vi "PreferencesLoop.vi"   [LabVIEW 2013]
panel:
  # "Test Subsystem"
  # "Other Subsystem"
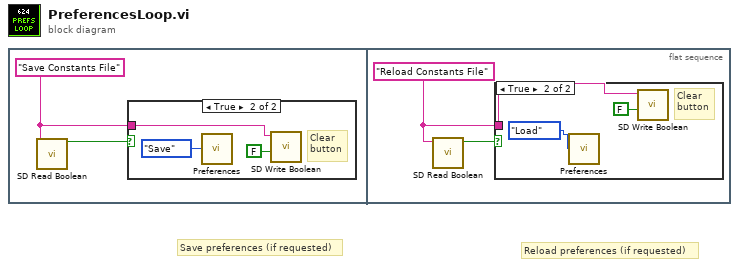
[diagram p0: block diagram]
diagram:
  # "Reload preferences (if requested)"
  # "Save preferences (if requested)"
  n1 = flat-sequence {
    frame #0 {
      w1 = "Save Constants File" ("Name")
      n2 = call <vilib>:"SD Read Boolean.vi"("Name"=w1) -> ("Boolean"=w2:bool)  [unwired: 8 in, 2 out]
      n3 = case shown="True" w2 {
        tunnel: w1 -> [_ w5]
        frame False {
          # "No update"
        }
        frame True {
          # "Clear\nbutton"
          n4 = call "Preferences.vi"("Operation"=enum16{"Load", "Save"}."Save") -> ()  [unwired: 1 in]
          n5 = call <vilib>:"SD Write Boolean.vi"("Boolean"=FALSE, "Name"=w5) -> ()  [unwired: 8 in, 2 out]
        }
      }
    }
    frame #1 {
      w7 = "Reload Constants File" ("Name")
      n6 = call <vilib>:"SD Read Boolean.vi"("Name"=w7) -> ("Boolean"=w6:bool)  [unwired: 8 in, 2 out]
      n7 = case shown="True" w6 {
        tunnel: w7 -> [_ w10]
        frame False {
          # "No update"
        }
        frame True {
          # "Clear\nbutton"
          n8 = call "Preferences.vi"("Operation"=enum16{"Load", "Save"}."Load") -> ()  [unwired: 1 in]
          n9 = call <vilib>:"SD Write Boolean.vi"("Boolean"=FALSE, "Name"=w10) -> ()  [unwired: 8 in, 2 out]
        }
      }
    }
  }
